vi "Result.Generate Xlink PN Init Report XML.vi"(4 "Name":string="Motor Jitter Test", 6 "Batch":string="Motor-Jitter-Test", 7 "Time Offset":dbl=-1.0, 8 "Folder":path, 9 "Operator":string, 10 "SN":string, 11 "StartTime":timestamp) -> (0 "error out":errorcluster, 3 "File Out":path)   [LabVIEW 2018]
panel:
  out "Data":string
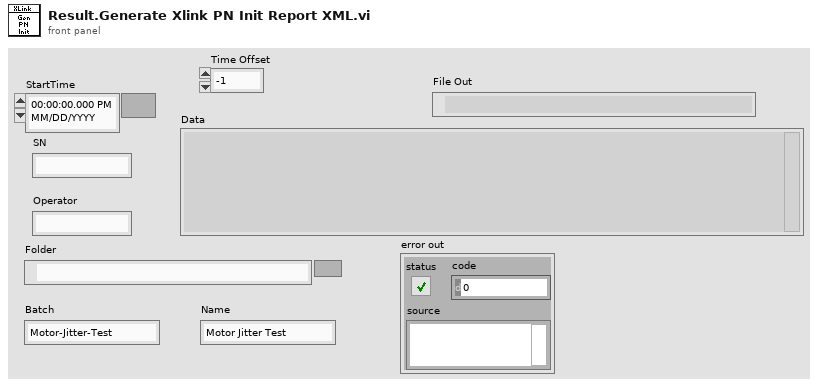
[diagram p1: front panel]
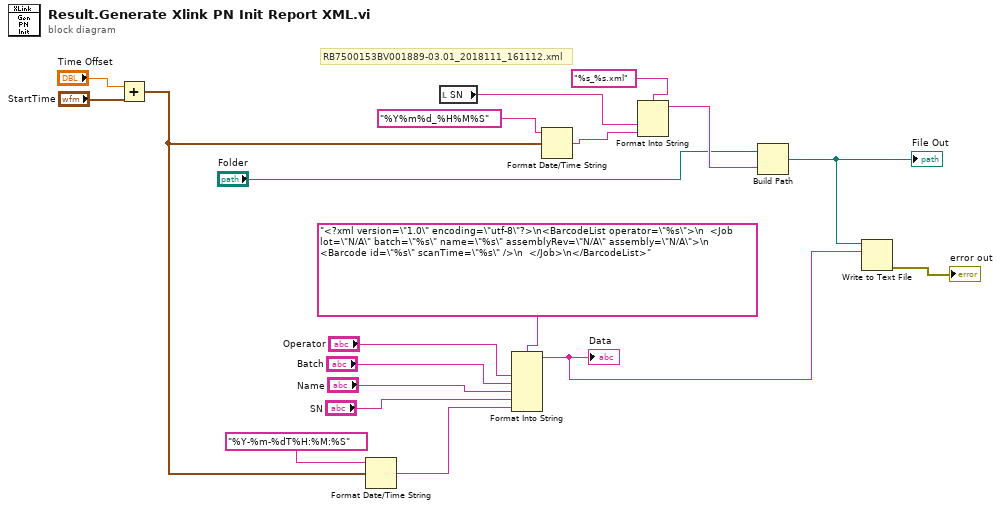
[diagram p0: block diagram]
diagram:
  # "RB7500153BV001889-03.01_2018111_161112.xml"
  n1 = Add(x="Time Offset", y="StartTime") -> (x+y=w1:timestamp)
  n2 = Format Date/Time String(time format string (%c)="%Y-%m-%dT%H:%M:%S", seconds (now)=w1) -> (date/time string=w13:string)  [unwired: 1 in]
  n3 = local read "SN"() -> (w11:string)
  n4 = Format Into String(format string="<?xml version=\"1.0\" encoding=\"utf-8\"?>\n<BarcodeList operator=\"%s\">\n  <Job lot=\"N/A\" batch=\"%s\" name=\"%s\" assemblyRev=\"N/A\" assembly=\"N/A\">\n    <Barcode id=\"%s\" scanTime=\"%s\" />\n  </Job>\n</BarcodeList>", "Operator", "Batch", "Name", "SN", w13) -> (resulting string=w12:string)  [unwired: 2 in, 1 out]
  "Data" <- w12
  n5 = Format Date/Time String(time format string (%c)="%Y%m%d_%H%M%S", seconds (now)=w1) -> (date/time string=w10:string)  [unwired: 1 in]
  n6 = Format Into String(format string="%s_%s.xml", w11, w10) -> (resulting string=w9:string)  [unwired: 2 in, 1 out]
  n7 = Build Path(base path="Folder", name or relative path=w9) -> (appended path=w7:path)
  "File Out" <- w7
  n8 = Write to Text File(file (use dialog)=w7, text=w12) -> (error out=→"error out":errorcluster)  [unwired: 2 in, 2 out]
